vi "K6485_I.vi"(1 "address":string="14") -> (0 "I":dbl=2.113269e-05 format="%.6e")   [LabVIEW 2021]
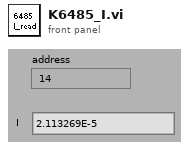
[diagram p1: front panel]
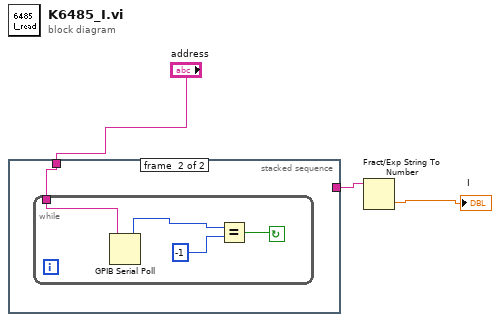
[diagram p0: block diagram]
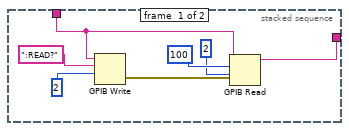
[diagram p2: hidden frame]
diagram:
  n1 = stacked-sequence {
    tunnel: "address" -> [w4 w11]
    tunnel: [w8 _] -> w1
    frame #0 {
      n2 = GPIB Write(0:w4, 1:":READ?", 2:2) -> (6:w5:errorcluster)  [unwired: 2 in, 1 out]
      n3 = GPIB Read(0:w4, 1:100, 2:2, 3:w5) -> (5:w8:string)  [unwired: 1 in, 2 out]
    }
    frame #1 {
      n4 = while {
        tunnel: w11 -> [w14]
        stop <- w15 continue-if-true
        n5 = GPIB Serial Poll(0:w14) -> (2:w13:i16)  [unwired: 1 in, 2 out]
        n6 = Equal?(x=w13, y=-1) -> (x = y?=w15:bool)
      }
    }
  }
  n7 = Fract/Exp String To Number(string=w1) -> (number=→"I":dbl)  [unwired: 3 in, 1 out]
